vi "taskTrialV1.vi"(6 "up or down":string, 7 "Rat ID":string, 8 "error in (no error)":errorcluster, 9 "previousChoices":i32[][](array[numeric]), 10 "Goal \nplatform":i32, 11 "Start \nplatform":i32) -> (0 "error out":errorcluster, 1 "previousChoices updated":i32[][](array[numeric]), 3 "choicesCurrent":i32[][](array[numeric]))   [LabVIEW 2017]
panel:
  out "Distance to goal":i32[](array[numeric])
  out "time":sgl
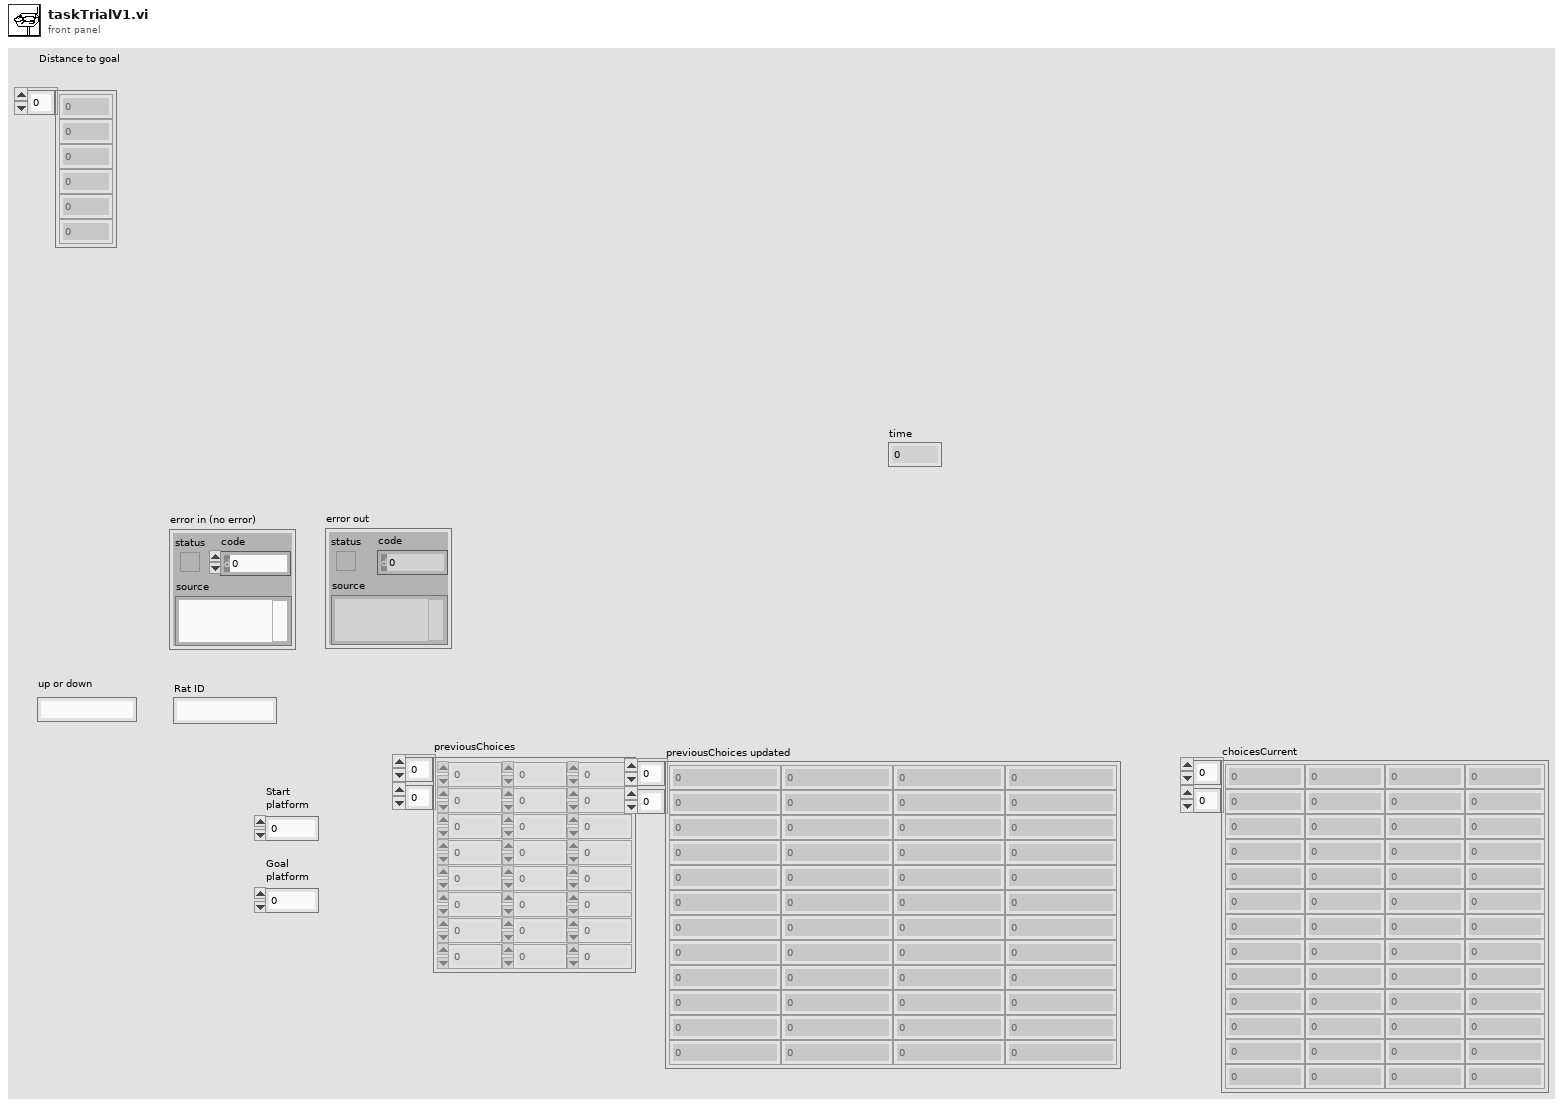
[diagram p1: front panel]
types:
  T1 = enum16{"open", "replace", "create", "open or create", "replace or create", "replace or create with confirmation"}
  T2 = enum16{"big-endian, network order", "native, host order", "little-endian"}
  T3 = cluster{"time":sgl, "Numeric":sgl, "Numeric":sgl, "Numeric":sgl}
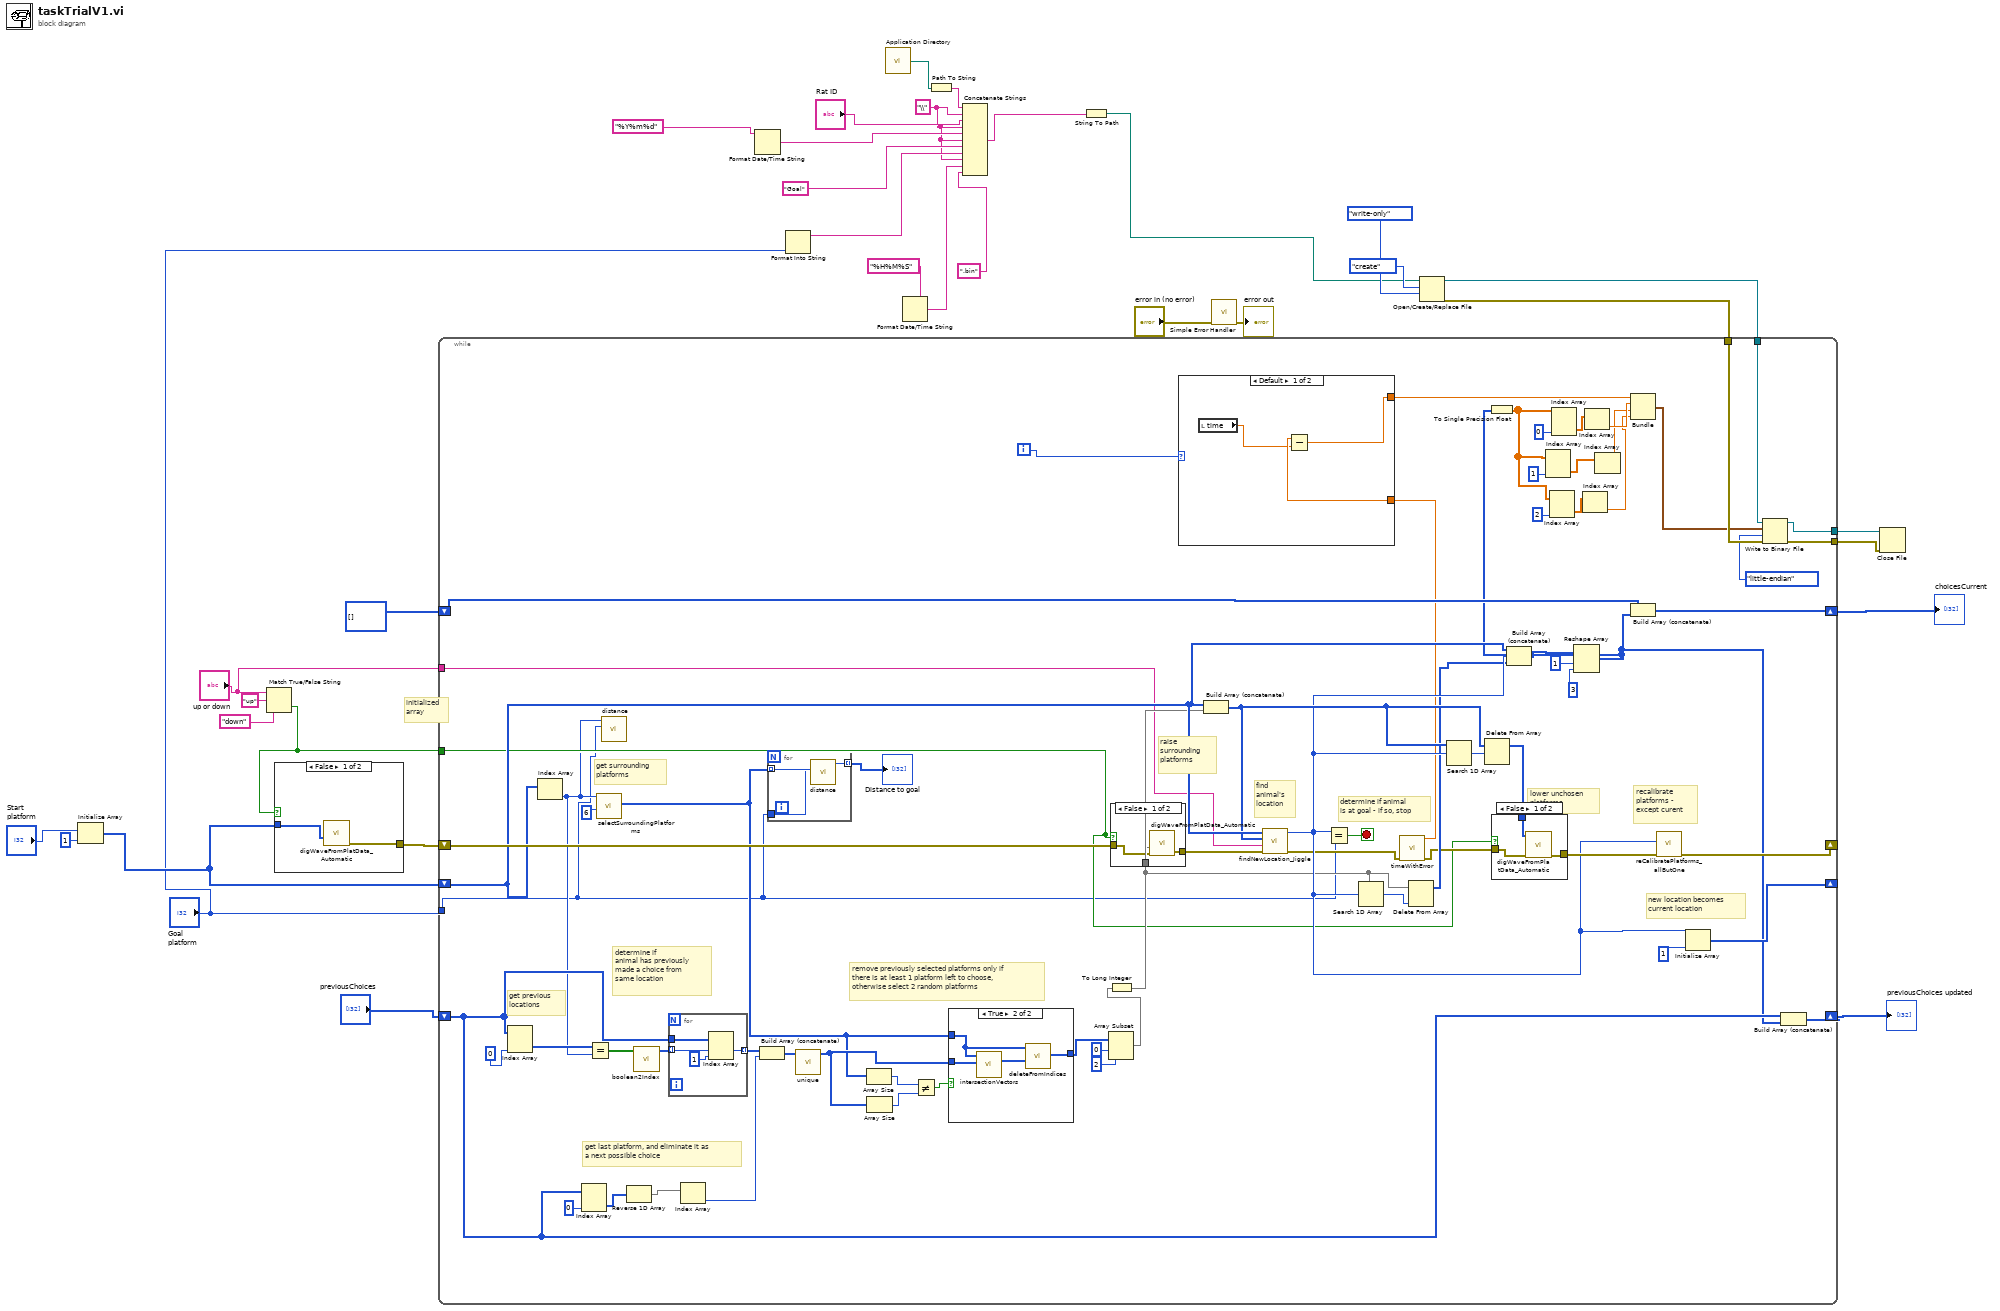
[diagram p0: block diagram]
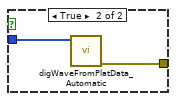
[diagram p2: hidden frame]
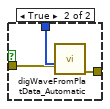
[diagram p3: hidden frame]
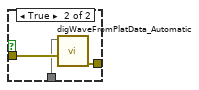
[diagram p4: hidden frame]
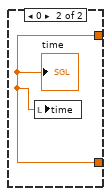
[diagram p5: hidden frame]
diagram:
  w9 = "\\" ("string")
  # "initialized\narray"
  n1 = Initialize Array("Start \nplatform", 1 ("dimension size")) -> (w26:i32[])
  n2 = Match True/False String(2:"down" ("false string"), 3:"up" ("true string"), 4:"up or down") -> (0:w2:bool)  [unwired: 1 out]
  n3 = case shown="False" w2 {
    tunnel: [w36 w38] -> w34
    tunnel: w26 -> [w35 w37]
    frame False {
      n4 = call "digWaveFromPlatData_Automatic.vi"("Platforms\nto lower"=w35) -> ("error out"=w36:errorcluster)  [unwired: 10 in]
    }
    frame True {
      n5 = call "digWaveFromPlatData_Automatic.vi"("Platforms\nto raise"=w37) -> ("error out"=w38:errorcluster)  [unwired: 10 in]
    }
  }
  n6 = Format Date/Time String(time format string (%c)="%Y%m%d" ("time string")) -> (date/time string=w11:string)  [unwired: 2 in]
  n7 = Format Into String("Goal \nplatform") -> (resulting string=w12:string)  [unwired: 3 in, 1 out]
  n8 = call <vilib>:"Application Directory.vi"() -> ("Application Directory"=w15:path)
  n9 = Format Date/Time String(time format string (%c)="%H%M%S" ("time string")) -> (date/time string=w7:string)  [unwired: 2 in]
  n10 = Path To String(path=w15) -> (string=w18:string)
  n11 = Concatenate Strings(w18, w9, "Rat ID", w9, w11, w9, "Goal" ("string"), w12, w9, w7, ".bin") -> (w5:string)
  n12 = String To Path(string=w5) -> (path=w14:path)
  n13 = call <vilib>:"Simple Error Handler.vi"("error in (no error)"="error in (no error)") -> ("error out"=→"error out":errorcluster)  [unwired: 4 in, 4 out]
  n14 = Open/Create/Replace File(file path (use dialog)=w14, operation (0:open)=T1."create", access (0:read/write)=enum16{"read/write", "read-only", "write-only"}."write-only") -> (refnum out=w22:refnum<file>, error out=w21:errorcluster)  [unwired: 3 in, 1 out]
  n15 = while {
    tunnel: "Goal \nplatform" -> [w39]
    shift-right: [w101] -> _
    shift-left: w34 -> [w100]
    shift-right: [w69] -> w32
    shift-left: i32[][] [] -> [w99]
    shift-right: [w88] -> w31
    shift-left: "previousChoices" -> [w77]
    shift-right: [w87] -> _
    shift-left: w26 -> [w82]
    tunnel: w22 -> [w66]
    tunnel: w21 -> [w65]
    tunnel: [w63] -> w20
    tunnel: [w62] -> w19
    tunnel: w2 -> [w44]
    tunnel: "up or down" -> [w43]
    i -> [w47]
    stop <- w104 stop-if-true
    # "get last platform, and eliminate it as \na next possible choice"
    # "determine if animal \nis at goal - if so, stop"
    # "remove previously selected platforms only if \nthere is at least 1 platform left to choose,\notherwise select 2 random platforms"
    # "determine if \nanimal has previously \nmade a choice from \nsame location"
    # "get previous \nlocations"
    # "get surrounding\nplatforms"
    # "new location becomes\ncurrent location"
    # "recalibrate \nplatforms - \nexcept curent"
    # "lower unchosen\nplatforms"
    # "find \nanimal's \nlocation"
    # "raise \nsurrounding \nplatforms"
    n16 = Index Array(array=w77, index (col)=0 ("disabled index (col)")) -> (element=w94:i32[])  [unwired: 1 in]
    n17 = Index Array(array=w82) -> (element=w40:i32)  [unwired: 1 in]
    n18 = Index Array(array=w77, index (col)=0 ("disabled index (col)")) -> (element=w79:i32[])  [unwired: 1 in]
    n19 = Equal?(x=w94, y=w40) -> (x = y?=w93:bool[])
    n20 = call "selectSurroundingPlatforms.vi"("Number of surrounding\nplatforms to raise"=6 ("Number of surrounding\nplatforms to raise"), "Start platform"=w40) -> ("Platforms \nto raise"=w41:i32[])  [unwired: 9 in]
    n21 = call "distance.vi"("Goal \nplatform"=w39, "Start \nplatform"=w40) -> ()  [unwired: 9 in, 1 out]
    n22 = Reverse 1D Array(array=w79) -> (reversed array=w78:i32[])
    n23 = call "boolean2Index.vi"("boolean"=w93) -> ("index"=w92:i32[])  [unwired: 10 in]
    n24 = for {
      tunnel: w92 -> [w134] mode=indexing
      tunnel: w77 -> [w135]
      tunnel: [w132] -> w76 mode=indexing
      n25 = Index Array(array=w135, index (row)=w134, index (col)=1) -> (element=w132:i32)
    }
    n26 = Index Array(array=w78) -> (element=w75:i32)  [unwired: 1 in]
    n27 = Build Array (concatenate)(w76, w75) -> (w74:i32[])
    n28 = for {
      tunnel: w41 -> [w110] mode=indexing
      tunnel: w39 -> [w109]
      tunnel: [w108] -> w42 mode=indexing
      n29 = call "distance.vi"("Goal \nplatform"=w109, "Start \nplatform"=w110) -> ("distance"=w108:i32)  [unwired: 9 in]
    }
    "Distance to goal" <- w42
    n30 = call "unique.vi"("Array"=w74) -> ("Array 2"=w73:i32[])  [unwired: 10 in]
    n31 = Array Size(array=w41) -> (size(s)=w85:i32)
    n32 = Array Size(array=w73) -> (size(s)=w84:i32)
    n33 = Not Equal?(x=w85, y=w84) -> (x != y?=w83:bool)
    n34 = case shown="True" w83 {
      tunnel: [w127 w130] -> w91
      tunnel: w41 -> [w127 w129]
      tunnel: w73 -> [_ w128]
      frame False {
      }
      frame True {
        n35 = call "intersectionVectors.vi"("vector2"=w128, "vector1"=w129) -> ("vector1 indices"=w131:i32[])  [unwired: 8 in, 1 out]
        n36 = call "deleteFromIndices.vi"("indices to delete"=w131, "vector"=w129) -> ("vector restricted"=w130:i32[])  [unwired: 9 in]
      }
    }
    n37 = Array Subset(array=w91, index=0, length=2) -> (w68:i32[])
    n38 = To Long Integer(number=w68) -> (32bit integer=w67:i32[])
    n39 = case shown="False" w44 {
      tunnel: w100 -> [w118 w122]
      tunnel: [w117 w121] -> w86
      tunnel: w67 -> [w119 w120]
      frame False {
        n40 = call "digWaveFromPlatData_Automatic.vi"("error in (no error)"=w118, "Platforms\nto lower"=w119) -> ("error out"=w117:errorcluster)  [unwired: 9 in]
      }
      frame True {
        n41 = call "digWaveFromPlatData_Automatic.vi"("error in (no error)"=w122, "Platforms\nto raise"=w120) -> ("error out"=w121:errorcluster)  [unwired: 9 in]
      }
    }
    n42 = Build Array (concatenate)(w82, w67) -> (w81:i32[])
    n43 = call "findNewLocation_Jiggle.vi"("error in (no error)"=w86, "up or down"=w43, "possible \nlocations"=w81, "start \nlocation"=w82) -> ("error out"=w48:errorcluster, "new\nplatform"=w72:i32)  [unwired: 6 in]
    n44 = Equal?(x=w72, y=w39) -> (x = y?=w104:bool)
    n45 = Search 1D Array(1D array=w67, element=w72) -> (index of element=w71:i32)  [unwired: 1 in]
    n46 = call "timeWithError.vi"("error in (no error)"=w48) -> ("time"=w45:sgl, "error out"=w49:errorcluster)  [unwired: 8 in]
    n47 = case shown="Default" w47 {
      tunnel: [w123 w126] -> w46
      tunnel: w45 -> [w125 w126]
      frame Default {
        n48 = local read "time"() -> (w124:sgl)
        n49 = Subtract(x=w125, y=w124) -> (x-y=w123:sgl)
      }
      frame 0 {
        n50 = local write "time"(w126) -> ()
        "time" <- w126
      }
    }
    n51 = Delete From Array(array=w67, index=w71) -> (array with subset deleted=w70:i32[])  [unwired: 1 in, 1 out]
    n52 = Search 1D Array(1D array=w81, element=w72) -> (index of element=w106:i32)  [unwired: 1 in]
    n53 = Delete From Array(array=w81, index=w106) -> (array with subset deleted=w105:i32[])  [unwired: 1 in, 1 out]
    n54 = case shown="False" w44 {
      tunnel: w105 -> [w113 w116]
      tunnel: [w111 w115] -> w102
      tunnel: w49 -> [w112 w114]
      frame False {
        n55 = call "digWaveFromPlatData_Automatic.vi"("error in (no error)"=w112, "Platforms\nto raise"=w113) -> ("error out"=w111:errorcluster)  [unwired: 9 in]
      }
      frame True {
        n56 = call "digWaveFromPlatData_Automatic.vi"("error in (no error)"=w114, "Platforms\nto lower"=w116) -> ("error out"=w115:errorcluster)  [unwired: 9 in]
      }
    }
    n57 = Build Array (concatenate)(w82, w72, w70) -> (w96:i32[])
    n58 = Reshape Array(w96, 1 ("dimension size"), 3 ("dimension size")) -> (w61:i32[][])
    n59 = To Single Precision Float(number=w61) -> (single precision float=w55:sgl[][])
    n60 = Index Array(array=w55, index (col)=1 ("disabled index (col)")) -> (element=w56:sgl[])  [unwired: 1 in]
    n61 = Index Array(array=w55, index (col)=2 ("disabled index (col)")) -> (element=w53:sgl[])  [unwired: 1 in]
    n62 = Index Array(array=w55, index (col)=0 ("disabled index (col)")) -> (element=w59:sgl[])  [unwired: 1 in]
    n63 = Index Array(array=w53) -> (element=w51:sgl)  [unwired: 1 in]
    n64 = Index Array(array=w59) -> (element=w58:sgl)  [unwired: 1 in]
    n65 = Index Array(array=w56) -> (element=w52:sgl)  [unwired: 1 in]
    n66 = Bundle("time"=w46, "Numeric"=w58, "Numeric"=w52, "Numeric"=w51) -> (w50:T3)  [unwired: 1 in]
    n67 = Build Array (concatenate)(w99, w61) -> (w69:i32[][])
    n68 = call "reCalibratePlatforms_allButOne.vi"("error in (no error)"=w102, "Current location"=w72) -> ("error out"=w101:errorcluster)  [unwired: 9 in]
    n69 = Initialize Array(w72, 1 ("dimension size")) -> (w87:i32[])
    n70 = Write to Binary File(file (use dialog)=w66, data=w50, error in=w65, 9:T2."little-endian" ("byte order (0:big-endian, network order)")) -> (refnum out=w63:refnum<file>, error out=w62:errorcluster)  [unwired: 2 in, 1 out]
    n71 = Build Array (concatenate)(w77, w61) -> (w88:i32[][])
  }
  "choicesCurrent" <- w32
  "previousChoices updated" <- w31
  n72 = Close File(refnum=w20, error in=w19) -> ()  [unwired: 2 out]
